vi "Handle Error.vi"(8 "error in":errorcluster, 11 "SCADA in":refnum<class "EMS.lvclass">) -> (0 "error out":errorcluster, 2 "stop actor?":bool=TRUE, 3 "SCADA out":refnum<class "EMS.lvclass">)   [LabVIEW 2018, in "EMS Core.lvlib" / "EMS.lvclass"]
doc: "(<B>Filename</B>: Actor Framework.lvlib:Actor.lvclass:Handle Error.vi)\n\nDefines how the actor handles an error that occurred while processing a message. By default, this method does nothing except stop the actor."
uses:
  EMS.lvclass
  EMS Generic Actor/EMS Generic/EMS Generic.lvclass
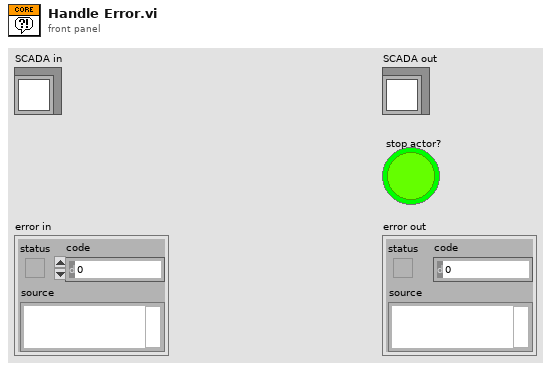
[diagram p1: front panel]
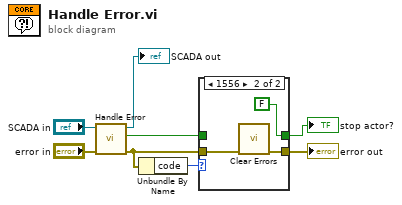
[diagram p0: block diagram]
diagram:
  n1 = call-parent "Handle Error.vi"("error in (no error)"="error in", "Actor in"="SCADA in") -> ("error out"=w4:errorcluster, "stop actor?"=w2:bool, "Actor out"=→"SCADA out":refnum<class "EMS.lvclass">)  [unwired: 7 in]
  n2 = Unbundle By Name(w4) -> ("code"=w5:i32)
  n3 = case shown="1556" w5 {
    tunnel: [w9 w11] -> w3
    tunnel: w4 -> [w9 w13]
    tunnel: [w10 FALSE ("stop actor?")] -> w1
    tunnel: w2 -> [w10 _]
    frame 0, Default {
    }
    frame 1556 {
      n4 = call <vilib>:"Clear Errors.vi"("error in (no error)"=w13) -> ("error out"=w11:errorcluster)  [unwired: 5 in, 1 out]
    }
  }
  "error out" <- w3
  "stop actor?" <- w1
